vi "例2.1数据流举例.vi"() -> ()   [LabVIEW 2012]
panel:
  out "结果2":dbl
  out "结果1":dbl
  in  "数值4":dbl
  in  "数值3":dbl
  in  "数值2":dbl
  in  "数值1":dbl
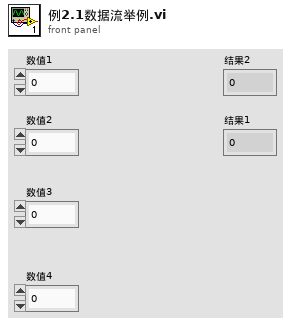
[diagram p1: front panel]
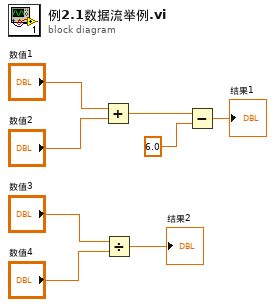
[diagram p0: block diagram]
diagram:
  n1 = Add(x="数值1", y="数值2") -> (x+y=w6:dbl)
  n2 = Divide(x="数值3", y="数值4") -> (x/y=→"结果2":dbl)
  n3 = Subtract(x=w6, y=6.0) -> (x-y=→"结果1":dbl)
